vi "Create Hardware Configuration UI.vi"(8 "error in (no error)":errorcluster, 11 "Path":path) -> (0 "error out":errorcluster, 3 "XML File Path(duplicate)":path)   [LabVIEW 2018]
uses:
  Resources/Type Defs/Shutter Configuration.ctl
  Resources/Type Defs/Stage Configuration.ctl
  Resources/Type Defs/Virtual Camera Configuration.ctl
  Resources/Type Defs/Camera Type.ctl
  Resources/Type Defs/Laser Configuration.ctl
  Resources/Type Defs/Physical Camera Assignment.ctl
  Resources/Type Defs/Microscope Configuration.ctl
  Resources/Type Defs/Microscope Type.ctl
  Resources/Type Defs/Hardware Configuration.ctl
  Resources/Type Defs/Pump Configuration.ctl
  <vilib>/Utility/xml.llb/Read From XML File(string).vi
  <vilib>/Utility/xml.llb/Write to XML File(string).vi
panel:
  in  "Cancel Button":bool
  in  "OK Button":bool
  in  "Microscope":T1={"Serial Port"="COM2", "Microscope Type"=enum."Ti2", "Detection Settings"=[{"Name"="Cy2 (Right)", "Filter Position"=1, "Optical Path"=2}, {"Name"="Cy3 (Right)", "Filter Position"=2, "Optical Path"=2}, {"Name"="Cy5 (Right)", "Filter Position"=3, "Optical Path"=2}, {"Name"="Cy7 (Right)", "Filter Position"=4, "Optical Path"=2}, {"Name"="No Filter (Right)", "Filter Position"=5, "Optical Path"=2}, {"Name"="Lasers to Eyes", "Filter Position"=6, "Optical Path"=1}]}
  in  "Cameras":T3[](array[typedef])=[{"Channel Name"="Cy2", "Camera Type"=enum."Hamamatsu", "Serial Number"="001790", "Flip Vertically"=FALSE, "Flip Horizontally"=TRUE, "photonsPerCount"=0.49, "wavelength"=473}, {"Channel Name"="Cy3", "Camera Type"=enum."Hamamatsu", "Serial Number"="740916", "Flip Vertically"=FALSE, "Flip Horizontally"=FALSE, "photonsPerCount"=0.5, "wavelength"=532}, {"Channel Name"="Cy5", "Camera Type"=enum."Hamamatsu", "Serial Number"="002242", "Flip Vertically"=FALSE, "Flip Horizontally"=FALSE, "photonsPerCount"=0.49, "wavelength"=640}, {"Channel Name"="Cy7", "Camera Type"=enum."Hamamatsu", "Serial Number"="002221", "Flip Vertically"=FALSE, "Flip Horizontally"=TRUE, "photonsPerCount"=0.49, "wavelength"=721}]
  in  "Lasers":T5[](array[typedef])=[{"Serial Port"="COM6", "Laser Type"=enum."Laser Quantum", "Polarizer Amplitude"=0.0, "Polarizer Theta Zero"=0.0, "Wavelength"=473}, {"Serial Port"="COM9", "Laser Type"=enum."Laser Quantum", "Polarizer Amplitude"=0.0, "Polarizer Theta Zero"=0.0, "Wavelength"=532}]
  in  "Camera Driver":T6={"Camera Type"=enum."Hamamatsu", "Sync Line"="Dev1/port2/line7"}
  in  "Stage":T7={"Serial Port"="COM4", "Forward Step (mm)"=0.4, "Lane Length (mm)"=6.0, "Lane Separation (mm)"=0.8, "Stage Type"=enum."ESP301"}
  in  "Shutters":T8[](array[typedef])=[{"IO Line"="Dev1/port1/line0", "Name"="Cy2", "Wavelength"=473, "Max rate (Hz)"=0.0}, {"IO Line"="Dev1/port1/line1", "Name"="Cy3", "Wavelength"=532, "Max rate (Hz)"=0.0}, {"IO Line"="Dev1/port1/line2", "Name"="Cy5", "Wavelength"=640, "Max rate (Hz)"=0.0}, {"IO Line"="Dev1/port1/line3", "Name"="Cy7", "Wavelength"=721, "Max rate (Hz)"=0.0}]
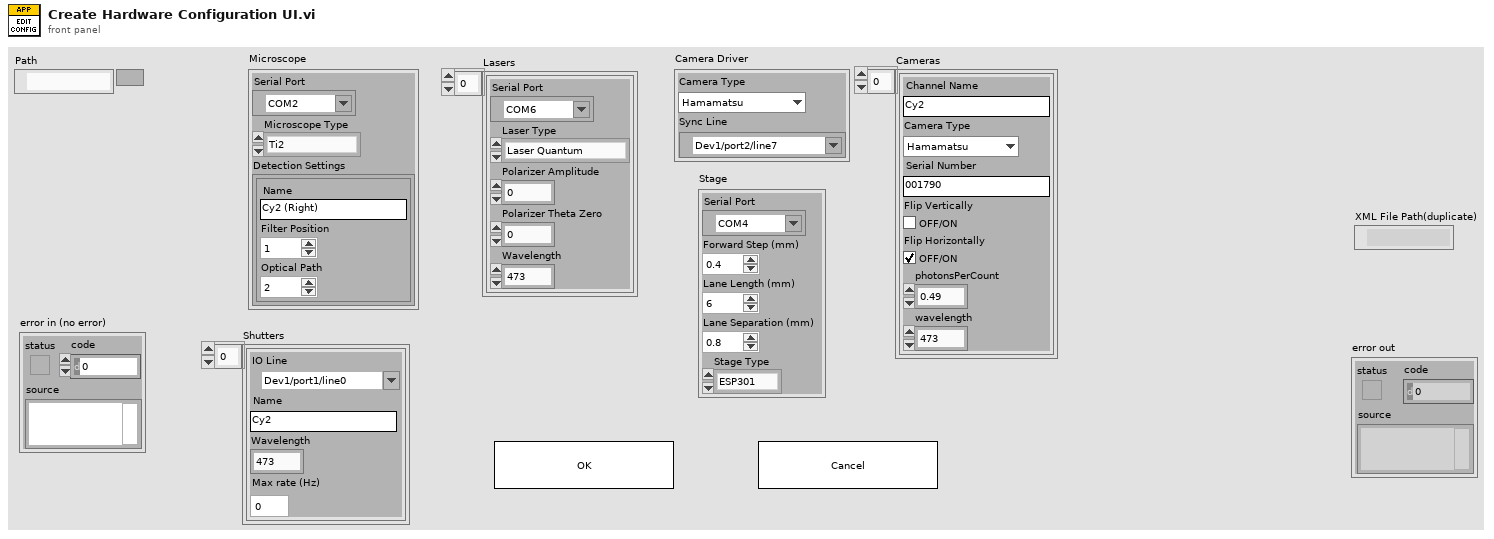
[diagram p1: front panel]
types:
  T1 = typedef "Microscope Configuration.ctl" = cluster{"Serial Port":refnum<visa-resource-name>, "Microscope Type":T2, "Detection Settings":cluster{"Name":string, "Filter Position":u16, "Optical Path":u16}[]}
  T2 = typedef "Microscope Type.ctl" = enum16{"Disable", "TE2000", "Eclipse Ti", "Ti2"}
  T3 = typedef "Physical Camera Assignment.ctl" = cluster{"Channel Name":string, "Camera Type":T4, "Serial Number":string, "Flip Vertically":bool, "Flip Horizontally":bool, "photonsPerCount":dbl, "wavelength":i16}
  T4 = typedef "Camera Type.ctl" = enum16{"Hamamatsu"}
  T5 = typedef "Laser Configuration.ctl" = cluster{"Serial Port":refnum<visa-resource-name>, "Laser Type":enum16{"Disable", "Laser Quantum", "Coherent OBIS", "PRM1-Z8"}, "Polarizer Amplitude":dbl, "Polarizer Theta Zero":dbl, "Wavelength":u16}
  T6 = typedef "Virtual Camera Configuration.ctl" = cluster{"Camera Type":T4, "Sync Line":tag}
  T7 = typedef "Stage Configuration.ctl" = cluster{"Serial Port":refnum<visa-resource-name>, "Forward Step (mm)":dbl, "Lane Length (mm)":dbl, "Lane Separation (mm)":dbl, "Stage Type":enum16{"Disabled", "ESP301", "Ti2"}}
  T8 = typedef "Shutter Configuration.ctl" = cluster{"IO Line":tag, "Name":string, "Wavelength":u16, "Max rate (Hz)":dbl}
  T9 = typedef "Hardware Configuration.ctl" = cluster{"Shutters":T8[], "Stage Configuration":T7, "Microscope Configuration":T1, "Virtual Camera Configuration":T6, "Laser Configuration":T5[], "Fluidics Configuration":T10, "Installed Cameras":T3[]}
  T10 = typedef "Pump Configuration.ctl" = cluster{"Fluidics present":bool}
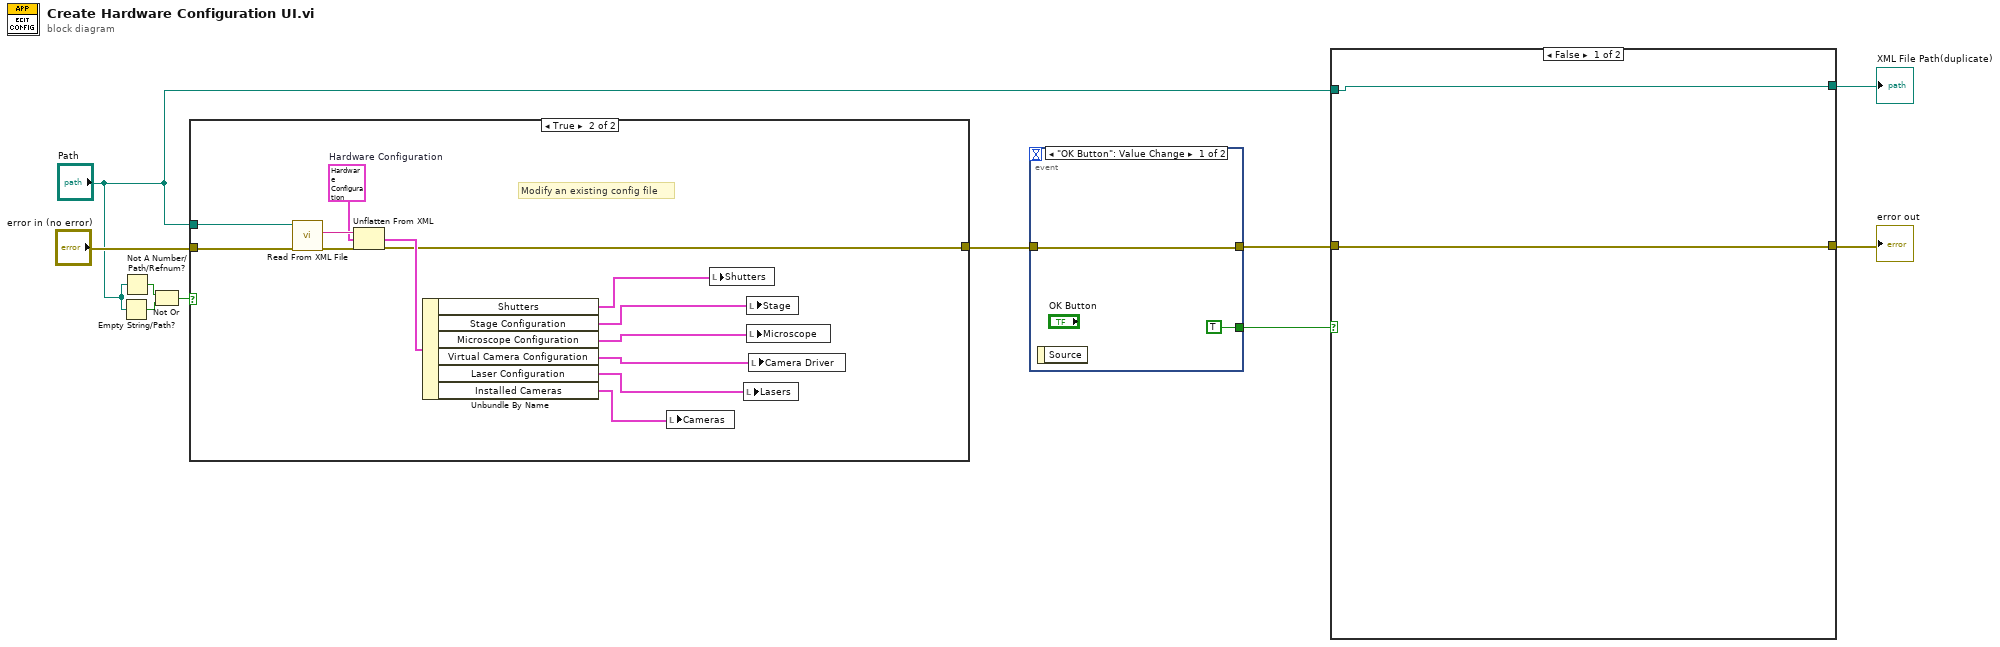
[diagram p0: block diagram]
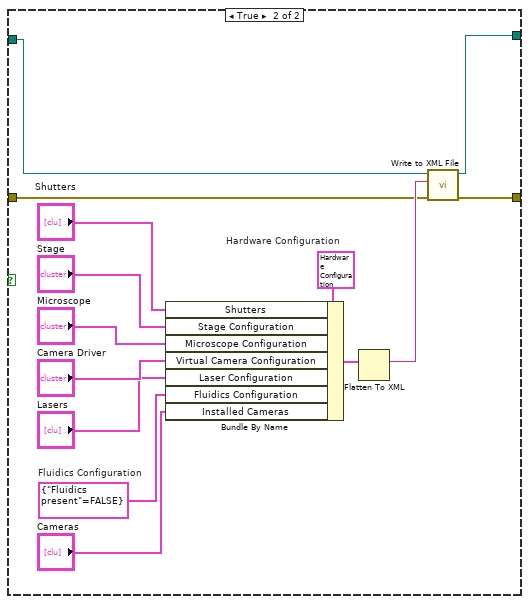
[diagram p2: hidden frame]
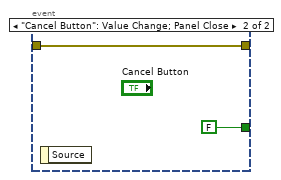
[diagram p3: hidden frame]
diagram:
  n1 = Empty String/Path?(string/path="Path") -> (empty?=w7:bool)
  n2 = Not A Number/Path/Refnum?(number/path/refnum="Path") -> (NaN/Path/Refnum?=w8:bool)
  n3 = Not Or(1:w7, 2:w8) -> (0:w9:bool)
  n4 = case shown="True" w9 {
    tunnel: "Path" -> [_ w24]
    tunnel: "error in (no error)" -> [w11 w21]
    tunnel: [w11 w12] -> w6
    frame False {
      # "Create a new config file"
    }
    frame True {
      w20 = T9 {"Shutters"=[], "Stage Configuration"={"Serial Port"="COM3", "Forward Step (mm)"=0.4, "Lane Length (mm)"=6.0, "Lane Separation (mm)"=0.8, "Stage Type"=enum."ESP301"}, "Microscope Configuration"={"Serial Port"="COM2", "Microscope Type"=enum."TE2000", "Detection Settings"=[]}, "Virtual Camera Configuration"={"Camera Type"=enum."Hamamatsu", "Sync Line"=""}, "Laser Configuration"=[], "Fluidics Configuration"={"Fluidics present"=FALSE}, "Installed Cameras"=[]}  # Hardware Configuration
      # "Modify an existing config file"
      n5 = call-poly <vilib>:"Read From XML File.vi"("error in (no error)"=w21, "XML File Path"=w24) -> ("error out"=w22:errorcluster, "XML Elements"=w23:string)  [unwired: 7 in, 1 out]
      n6 = Unflatten From XML(xml string=w23, type=w20, error in (no error)=w22) -> (value=w19:T9, error out=w12:errorcluster)
      n7 = Unbundle By Name(w19) -> ("Shutters"=w18:T8[], "Stage Configuration"=w17:T7, "Microscope Configuration"=w16:T1, "Virtual Camera Configuration"=w15:T6, "Laser Configuration"=w14:T5[], "Installed Cameras"=w13:T3[])
      n8 = local write "Cameras"(w13) -> ()
      n9 = local write "Shutters"(w18) -> ()
      n10 = local write "Lasers"(w14) -> ()
      n11 = local write "Stage"(w17) -> ()
      n12 = local write "Microscope"(w16) -> ()
      n13 = local write "Camera Driver"(w15) -> ()
    }
  }
  n14 = event shown="[0] \"OK Button\": Value Change" {
    selector: _ -> [_ _]
    dyn-events: _ -> [_ _]
    timeout: _ -> [_ _]
    tunnel: w6 -> [w26 w27]
    tunnel: [w26 w27] -> w5
    tunnel: [TRUE FALSE] -> w4
    event "OK Button": Value Change {
      n15 = event-data() -> ()  [unwired: 1 in, 1 out]
    }
    event "Cancel Button": Value Change; Panel Close {
      n16 = event-data() -> ()  [unwired: 1 in, 1 out]
    }
  }
  n17 = case shown="False" w4 {
    tunnel: w5 -> [w30 w34]
    tunnel: "Path" -> [w29 w33]
    tunnel: [w30 w32] -> w2
    tunnel: [w29 w31] -> w1
    frame False {
    }
    frame True {
      w37 = T9 {"Shutters"=[], "Stage Configuration"={"Serial Port"="COM3", "Forward Step (mm)"=0.4, "Lane Length (mm)"=6.0, "Lane Separation (mm)"=0.8, "Stage Type"=enum."ESP301"}, "Microscope Configuration"={"Serial Port"="COM2", "Microscope Type"=enum."TE2000", "Detection Settings"=[]}, "Virtual Camera Configuration"={"Camera Type"=enum."Hamamatsu", "Sync Line"=""}, "Laser Configuration"=[], "Fluidics Configuration"={"Fluidics present"=FALSE}, "Installed Cameras"=[]}  # Hardware Configuration
      w38 = T10 {"Fluidics present"=FALSE}  # Fluidics Configuration
      n18 = Bundle By Name(cluster=w37, "Shutters"="Shutters", "Stage Configuration"="Stage", "Microscope Configuration"="Microscope", "Virtual Camera Configuration"="Camera Driver", "Laser Configuration"="Lasers", "Fluidics Configuration"=w38, "Installed Cameras"="Cameras") -> (w44:T9)
      n19 = Flatten To XML(anything=w44) -> (xml string=w39:string)
      n20 = call-poly <vilib>:"Write to XML File.vi"("error in (no error)"=w34, "XML Input"=w39, "XML File Path"=w33) -> ("error out"=w32:errorcluster, "XML File Path(duplicate)"=w31:path)  [unwired: 6 in, 1 out]
    }
  }
  "error out" <- w2
  "XML File Path(duplicate)" <- w1
